vi "SetAndorOnlineOfflineFGV.vi"(8 "error in":errorcluster, 9 "andor 2":bool=TRUE, 10 "Set_Get":enum16{"Set", "Get"}(ring), 11 "andor 0":bool=TRUE) -> (0 "error out":errorcluster, 2 "andor 1":bool, 3 "andor 0":bool)   [LabVIEW 2010]
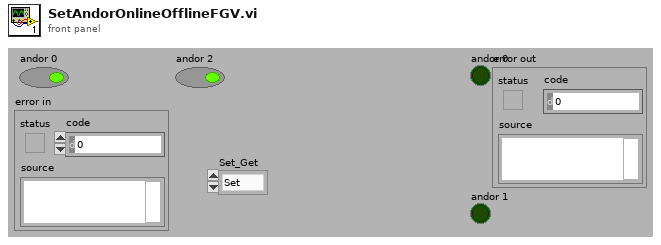
[diagram p1: front panel]
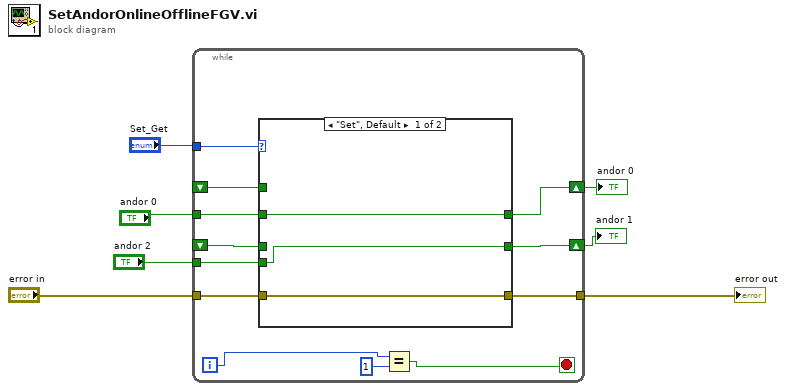
[diagram p0: block diagram]
diagram:
  n1 = while {
    tunnel: "Set_Get" -> [w19]
    tunnel: "andor 0" -> [w18]
    shift-right: [w17] -> w5
    shift-left: _ -> [w16]
    tunnel: "error in" -> [w12]
    tunnel: [w11] -> w3
    shift-right: [w10] -> w2
    shift-left: _ -> [w9]
    tunnel: "andor 2" -> [w8]
    i -> [w13]
    stop <- w14 stop-if-true
    n2 = case shown="\"Set\", Default" w19 {
      tunnel: w18 -> [w22 _]
      tunnel: [w22 w25] -> w17
      tunnel: w16 -> [_ w25]
      tunnel: [w21 w24] -> w11
      tunnel: w12 -> [w21 w24]
      tunnel: [w20 w23] -> w10
      tunnel: w9 -> [_ w23]
      tunnel: w8 -> [w20 _]
      frame "Set", Default {
      }
      frame "Get" {
      }
    }
    n3 = Equal?(x=w13, y=1) -> (x = y?=w14:bool)
  }
  "andor 0" <- w5
  "error out" <- w3
  "andor 1" <- w2
